vi "Update Status.vi"(8 "error in (no error)":errorcluster, 10 "Status":string, 11 "Person In":refnum<class "Person.lvclass">) -> (0 "error out":errorcluster, 3 "Person Out":refnum<class "Person.lvclass">)   [LabVIEW 2020, in "Person.lvclass"]
uses:
  Person.lvclass
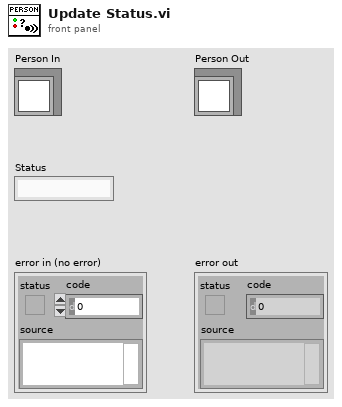
[diagram p1: front panel]
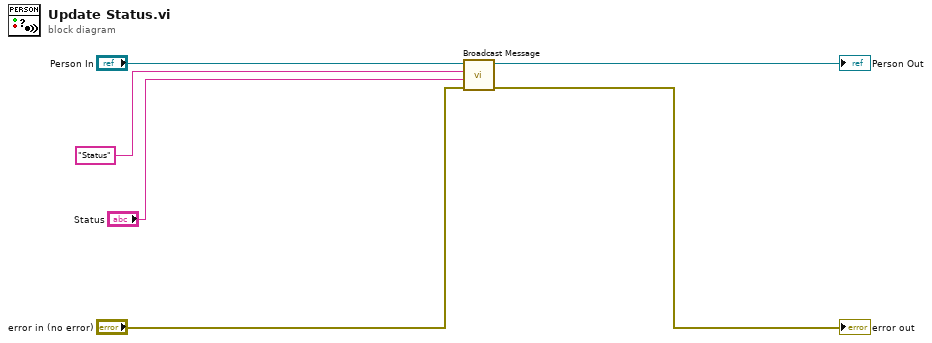
[diagram p0: block diagram]
diagram:
  n1 = call-dynamic "Broadcast Message.vi"("error in (no error)"="error in (no error)", "Message Data"="Status", "Message"="Status", "Rig Process In"="Person In") -> ("error out"=→"error out":errorcluster, "Rig Process Out"=→"Person Out":refnum<class "Person.lvclass">)  [unwired: 6 in]
